vi "TestModule.vi"(10 "test module":T1, 11 "IA State":T3={"our_robots"=[], "enemy_robots"=[], "balls"=[], "geometry"={"field_length"=0, "field_width"=0, "goal_width"=0, "goal_depth"=0, "center_circle_radius"=0, "defense_width"=0, "defense_depth"=0, "free_kick_from_defense_dist"=0, "penalty_spot_from_field_line_dist"=0, "penalty_line_from_spot_dist"=0, "half_moon_depth"=0, "half_moon_width"=0}, "IA Judge"={"stage"="", "command"="", "our_goalie_id"=0.0, "enemy_goalie_id"=0.0, "command enum"=enum."Halt", "Time"=enum."Azul"}, "Received Timestamp"=timestamp(0 s since 1904-01-01), "Events"={"Touch"=FALSE, "id touch"=0.0, "Ball out of \nVision"=FALSE, "Ball inside \nGoalie area"=FALSE, "Robot not responding"=FALSE, "Robots responding status"=[1.0, 1.0, 1.0, 1.0, 1.0, 1.0], "Enemy Ball \nPossession"=FALSE, "Id ini Possession"=0.0, "Ball Possesion"=FALSE, "Id Possesion"=0.0, "Ball at\nour goal side"=FALSE, "Ball at\ntouchline"=FALSE, "Ball at\nenemy goal side"=FALSE}}) -> (3 "output cluster IA":T3={"our_robots"=[], "enemy_robots"=[], "balls"=[], "geometry"={"field_length"=0, "field_width"=0, "goal_width"=0, "goal_depth"=0, "center_circle_radius"=0, "defense_width"=0, "defense_depth"=0, "free_kick_from_defense_dist"=0, "penalty_spot_from_field_line_dist"=0, "penalty_line_from_spot_dist"=0, "half_moon_depth"=0, "half_moon_width"=0}, "IA Judge"={"stage"="", "command"="", "our_goalie_id"=0.0, "enemy_goalie_id"=0.0, "command enum"=enum."Halt", "Time"=enum."Azul"}, "Received Timestamp"=timestamp(0 s since 1904-01-01), "Events"={"Touch"=FALSE, "id touch"=0.0, "Ball out of \nVision"=FALSE, "Ball inside \nGoalie area"=FALSE, "Robot not responding"=FALSE, "Robots responding status"=[1.0, 1.0, 1.0, 1.0, 1.0, 1.0], "Enemy Ball \nPossession"=FALSE, "Id ini Possession"=0.0, "Ball Possesion"=FALSE, "Id Possesion"=0.0, "Ball at\nour goal side"=FALSE, "Ball at\ntouchline"=FALSE, "Ball at\nenemy goal side"=FALSE}})   [LabVIEW 2018]
uses:
  Core/AI Input.ctl
  Core/AI Robot.ctl
  Functions Enum.ctl
  AttackerStates.ctl
  Path Planning/RRT/PathDests.ctl
  Path Planning/RRT/PathDest.ctl
  Core/AI Ball.ctl
  Core/Field Size.ctl
  Core/AI Judge.ctl
  Command Enum.ctl
  Util/Events/Events.ctl
  Test/TestModule.ctl
  Util/Select None or Robot.ctl
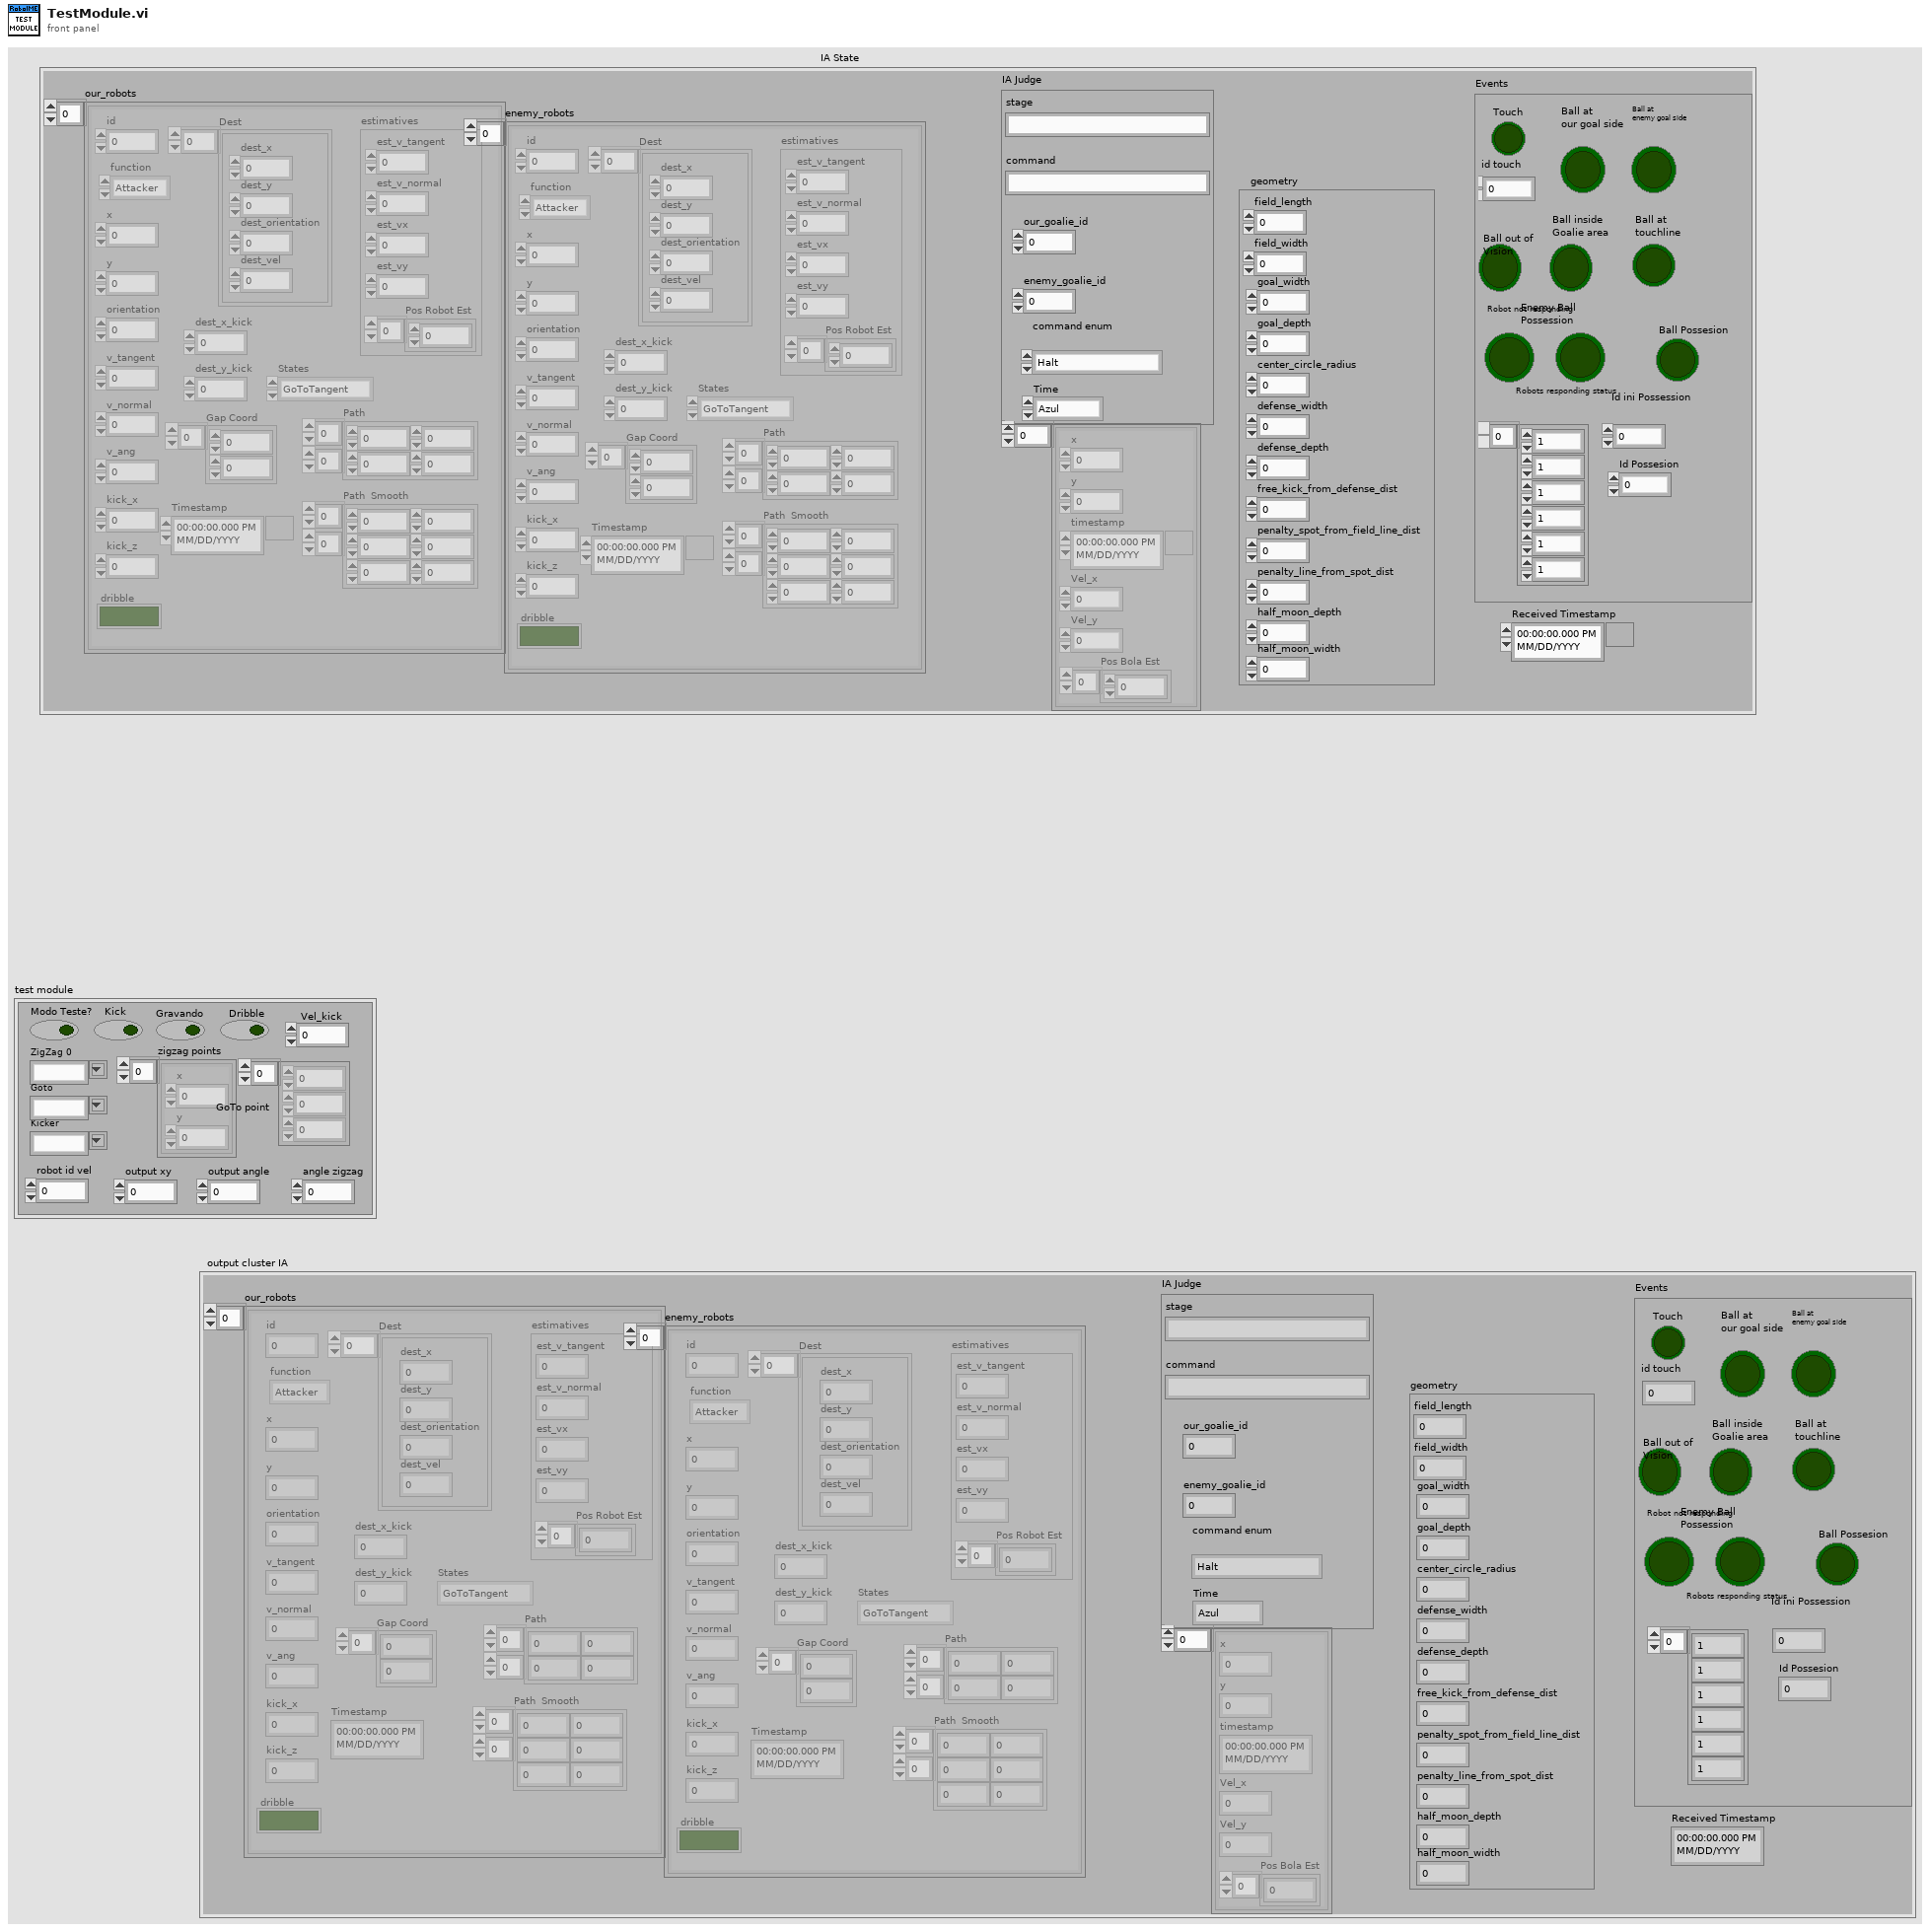
[diagram p1: front panel]
types:
  T1 = typedef "TestModule.ctl" = cluster{"Goto":T2, "ZigZag 0":T2, "Kicker":T2, "Vel_kick":dbl, "Kick":bool, "Modo Teste?":bool, "GoTo point":dbl[], "zigzag points":cluster{"x":dbl, "y":dbl}[], "robot id vel":u32, "Dribble":bool, "Gravando":bool, "output xy":dbl, "output angle":dbl, "angle zigzag":dbl}
  T2 = typedef "Select None or Robot.ctl" = string
  T3 = typedef "AI Input.ctl" = cluster{"our_robots":T4[], "enemy_robots":T4[], "balls":T9[], "geometry":T10, "IA Judge":T11, "Received Timestamp":timestamp, "Events":T13}
  T4 = typedef "AI Robot.ctl" = cluster{"id":u32, "function":T5, "x":dbl, "y":dbl, "orientation":dbl, "v_tangent":dbl, "v_normal":dbl, "v_ang":dbl, "kick_x":dbl, "kick_z":dbl, "dribble":bool, "Timestamp":timestamp, "estimatives":cluster{"est_v_tangent":dbl, "est_v_normal":dbl, "est_vx":dbl, "est_vy":dbl, "Pos Robot Est":dbl[]}, "dest_x_kick":dbl, "dest_y_kick":dbl, "Gap Coord":dbl[], "States":T6, "Path ":dbl[][], "Path  Smooth":dbl[][], "Dest":T7}
  T5 = typedef "Functions Enum.ctl" = enum16{"Attacker", "Goalie", "Defender", "Striker", "Goto 0", "Dummy", "Kicker", "ZigZag"}
  T6 = typedef "AttackerStates.ctl" = enum16{"Pass", "GoToTangent", "BallGetting", "GoToKick", "Rotate anti-clockwise", "Rotate Clockwise", ""}
  T7 = typedef "PathDests.ctl" = T8[]
  T8 = typedef "PathDest.ctl" = cluster{"dest_x":dbl, "dest_y":dbl, "dest_orientation":dbl, "dest_vel":dbl}
  T9 = typedef "AI Ball.ctl" = cluster{"x":dbl, "y":dbl, "timestamp":timestamp, "Vel_x":dbl, "Vel_y":dbl, "Pos Bola Est":dbl[]}
  T10 = typedef "Field Size.ctl" = cluster{"field_length":u32, "field_width":u32, "goal_width":u32, "goal_depth":u32, "center_circle_radius":u32, "defense_width":u32, "defense_depth":u32, "free_kick_from_defense_dist":u32, "penalty_spot_from_field_line_dist":u32, "penalty_line_from_spot_dist":u32, "half_moon_depth":u32, "half_moon_width":u32}
  T11 = typedef "AI Judge.ctl" = cluster{"stage":string, "command":string, "our_goalie_id":dbl, "enemy_goalie_id":dbl, "command enum":T12, "Time":enum16{"Azul", "Amarelo"}}
  T12 = typedef "Command Enum.ctl" = enum16{"Halt", "Stop", "Force Start", "PKA Normal Start", "Prepare Kickoff Ally", "PKE Normal Start", "Prepare Kickoff Enemy", "Prepare Penalty Ally", "PPA Normal Start", "Prepare Penalty Enemy", "PPE Normal Start", "Ball Placement Enemy Up", "Ball Placement Enemy Down", "Ball Placement Ally Up", "Ball Placement Ally Mid", "Ball Placement Ally Down", "Indirect Free Enemy", "Indirect Free Ally", "Timeout Enemy", "Timeout Ally", "Goal Enemy", "Goal Ally", "Normal Half Time", "Extra Time Break", "Extra Half Time", "None", "Post Game"}
  T13 = typedef "Events.ctl" = cluster{"Touch":bool, "id touch":dbl, "Ball out of \nVision":bool, "Ball inside \nGoalie area":bool, "Robot not responding":bool, "Robots responding status":dbl[], "Enemy Ball \nPossession":bool, "Id ini Possession":dbl, "Ball Possesion":bool, "Id Possesion":dbl, "Ball at\nour goal side":bool, "Ball at\ntouchline":bool, "Ball at\nenemy goal side":bool}
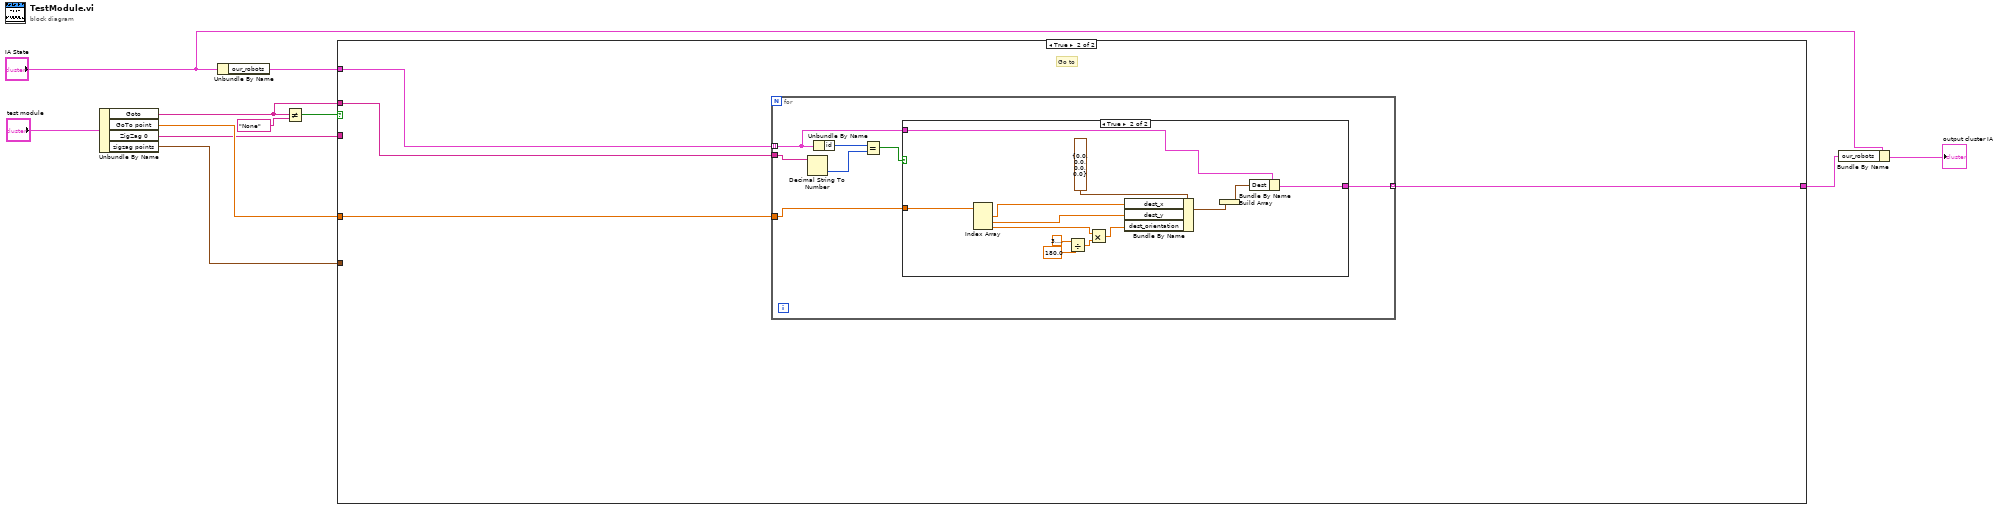
[diagram p0: block diagram]
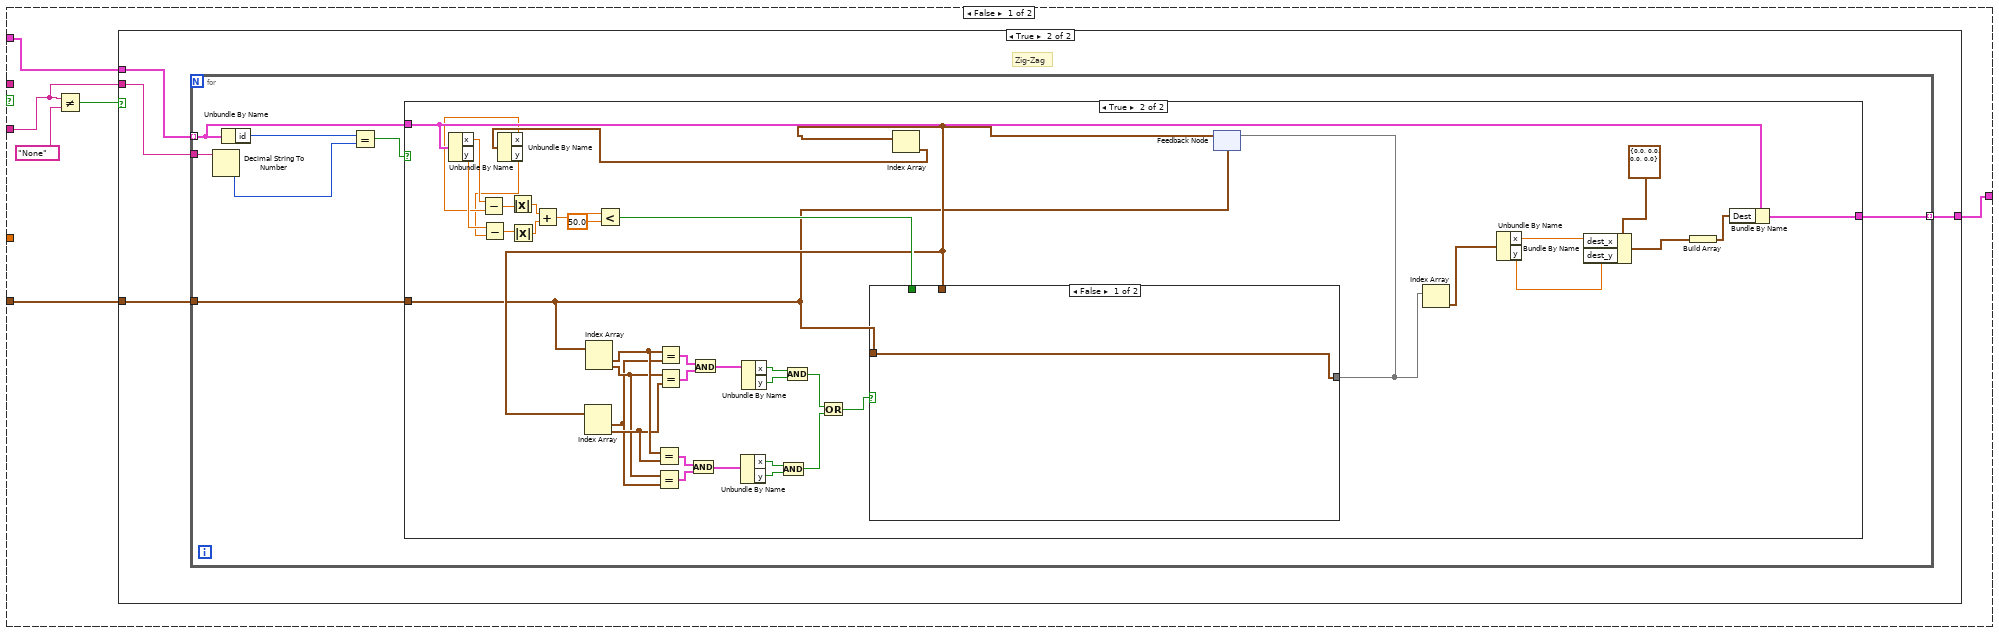
[diagram p2: hidden frame]
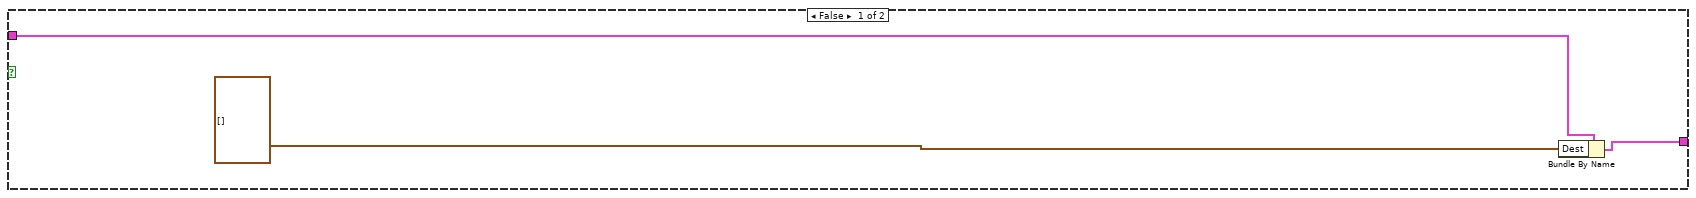
[diagram p4: hidden frame]
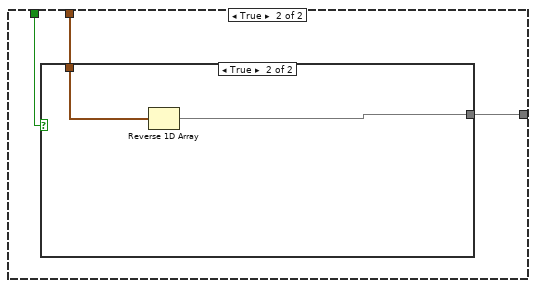
[diagram p5: hidden frame]
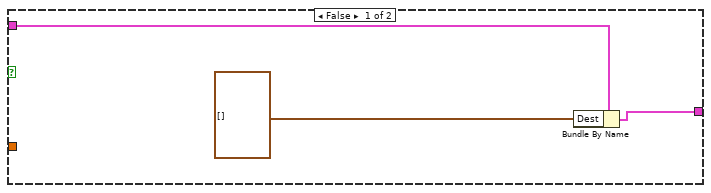
[diagram p7: hidden frame]
diagram:
  n1 = Unbundle By Name("test module") -> ("Goto"=w7:T2, "GoTo point"=w4:dbl[], "ZigZag 0"=w3:T2, "zigzag points"=w1:cluster{"x":dbl, "y":dbl}[])
  n2 = Unbundle By Name("IA State") -> ("our_robots"=w8:T4[])
  n3 = Not Equal?(x=w7, y=T2 "None") -> (x != y?=w9:bool)
  n4 = case shown="True" w9 {
    tunnel: w8 -> [w15 w83]
    tunnel: w7 -> [_ w82]
    tunnel: [w13 w81] -> w5
    tunnel: w4 -> [_ w80]
    tunnel: w3 -> [w14 _]
    tunnel: w1 -> [w12 _]
    frame False {
      n5 = Not Equal?(x=w14, y=T2 "None") -> (x != y?=w16:bool)
      n6 = case shown="True" w16 {
        tunnel: w15 -> [w18 w22]
        tunnel: w14 -> [_ w21]
        tunnel: [w18 w20] -> w13
        tunnel: w12 -> [_ w19]
        frame False {
          # "Test module sem comando"
        }
        frame True {
          # "Zig-Zag"
          n7 = for {
            tunnel: w22 -> [w25] mode=indexing
            tunnel: w21 -> [w26]
            tunnel: [w24] -> w20 mode=indexing
            tunnel: w19 -> [w23]
            n8 = Decimal String To Number(string=w26) -> (number=w29:i32)  [unwired: 2 in, 1 out]
            n9 = Unbundle By Name(w25) -> ("id"=w27:u32)
            n10 = Equal?(x=w27, y=w29) -> (x = y?=w28:bool)
            n11 = case shown="True" w28 {
              tunnel: [w31 w71] -> w24
              tunnel: w25 -> [w30 w68]
              tunnel: w23 -> [_ w50]
              frame False {
                n12 = Bundle By Name(cluster=w30, "Dest"=T7 []) -> (w31:T4)
              }
              frame True {
                n13 = Unbundle By Name(w68) -> ("x"=w63:dbl, "y"=w62:dbl)
                n14 = Index Array(array=w50) -> (element #1=w45:cluster{"x":dbl, "y":dbl}, element #2=w43:cluster{"x":dbl, "y":dbl})  [unwired: 2 in]
                n15 = feedback #1(w50) -> (w51:cluster{"x":dbl, "y":dbl}[])
                n16 = Index Array(array=w51) -> (element #1=w42:cluster{"x":dbl, "y":dbl}, element #2=w44:cluster{"x":dbl, "y":dbl})  [unwired: 2 in]
                n17 = Equal?(x=w45, y=w44) -> (x = y?=w46:cluster{"x":bool, "y":bool})
                n18 = Equal?(x=w43, y=w42) -> (x = y?=w47:cluster{"x":bool, "y":bool})
                n19 = Equal?(x=w45, y=w42) -> (x = y?=w49:cluster{"x":bool, "y":bool})
                n20 = Equal?(x=w43, y=w44) -> (x = y?=w48:cluster{"x":bool, "y":bool})
                n21 = And(x=w46, y=w47) -> (x .and. y?=w40:cluster{"x":bool, "y":bool})
                n22 = And(x=w49, y=w48) -> (x .and. y?=w41:cluster{"x":bool, "y":bool})
                n23 = Unbundle By Name(w40) -> ("x"=w37:bool, "y"=w36:bool)
                n24 = Unbundle By Name(w41) -> ("x"=w39:bool, "y"=w38:bool)
                n25 = And(x=w37, y=w36) -> (x .and. y?=w34:bool)
                n26 = And(x=w39, y=w38) -> (x .and. y?=w35:bool)
                n27 = Or(x=w35, y=w34) -> (x .or. y?=w33:bool)
                n28 = Index Array(array=w51) -> (element=w56:cluster{"x":dbl, "y":dbl})  [unwired: 1 in]
                n29 = Unbundle By Name(w56) -> ("x"=w55:dbl, "y"=w54:dbl)
                n30 = Subtract(x=w63, y=w55) -> (x-y=w67:dbl)
                n31 = Subtract(x=w62, y=w54) -> (x-y=w66:dbl)
                n32 = Absolute Value(x=w67) -> (abs(x)=w65:dbl)
                n33 = Absolute Value(x=w66) -> (abs(x)=w64:dbl)
                n34 = Add(x=w65, y=w64) -> (x+y=w61:dbl)
                n35 = Less?(x=w61, y=50.0) -> (x < y?=w59:bool)
                n36 = case shown="False" w33 {
                  tunnel: w59 -> [_ w76]
                  tunnel: [w73 w75] -> w57
                  tunnel: w51 -> [_ w74]
                  tunnel: w50 -> [w73 _]
                  frame False {
                  }
                  frame True {
                    n37 = case shown="True" w76 {
                      tunnel: [w77 w78] -> w75
                      tunnel: w74 -> [w77 w79]
                      frame False {
                      }
                      frame True {
                        n38 = Reverse 1D Array(array=w79) -> (reversed array=w78:cluster{"x":dbl, "y":dbl}[])
                      }
                    }
                  }
                }
                n39 = feedback-in #1(w57) -> ()
                n40 = Index Array(array=w57) -> (element=w58:cluster{"x":dbl, "y":dbl})  [unwired: 1 in]
                n41 = Unbundle By Name(w58) -> ("x"=w53:dbl, "y"=w52:dbl)
                n42 = Bundle By Name(cluster=T8 {"dest_x"=0.0, "dest_y"=0.0, "dest_orientation"=0.0, "dest_vel"=0.0} ("element"), "dest_x"=w53, "dest_y"=w52) -> (w69:T8)
                n43 = Build Array(w69) -> (w70:T8[])
                n44 = Bundle By Name(cluster=w68, "Dest"=w70) -> (w71:T4)
              }
            }
          }
        }
      }
    }
    frame True {
      # "Go to"
      n45 = for {
        tunnel: w83 -> [w86] mode=indexing
        tunnel: w82 -> [w89]
        tunnel: [w85] -> w81 mode=indexing
        tunnel: w80 -> [w84]
        n46 = Decimal String To Number(string=w89) -> (number=w88:i32)  [unwired: 2 in, 1 out]
        n47 = Unbundle By Name(w86) -> ("id"=w90:u32)
        n48 = Equal?(x=w90, y=w88) -> (x = y?=w87:bool)
        n49 = case shown="True" w87 {
          tunnel: w86 -> [w92 w106]
          tunnel: [w91 w102] -> w85
          tunnel: w84 -> [_ w101]
          frame False {
            n50 = Bundle By Name(cluster=w92, "Dest"=T7 []) -> (w91:T4)
          }
          frame True {
            n51 = Index Array(array=w101) -> (element #1=w100:dbl, element #2=w99:dbl, element #3=w95:dbl)  [unwired: 3 in]
            n52 = Divide(x=3.141592653589793, y=180.0) -> (x/y=w96:dbl)
            n53 = Multiply(x=w95, y=w96) -> (x*y=w94:dbl)
            n54 = Bundle By Name(cluster=T8 {"dest_x"=0.0, "dest_y"=0.0, "dest_orientation"=0.0, "dest_vel"=0.0} ("element"), "dest_x"=w100, "dest_y"=w99, "dest_orientation"=w94) -> (w104:T8)
            n55 = Build Array(w104) -> (w105:T8[])
            n56 = Bundle By Name(cluster=w106, "Dest"=w105) -> (w102:T4)
          }
        }
      }
    }
  }
  n57 = Bundle By Name(cluster="IA State", "our_robots"=w5) -> (→"output cluster IA":T3)
